vi "Goal_Clamp_on_Move.vi"(10 "Numeric":i32, 11 "60 Goal?":bool) -> ()   [LabVIEW 2012, in "Serenity_mk2.lvrbt"]
uses:
  Serenity_mk2.lvrbt
  <vilib>/NXT/Hardware/Plugins/Tetrix 180 deg Servo/Tetrix180ServoAddress.ctl
  <vilib>/NXT/NXTIO Xnodes/NXTIONodeSubVIs/TETRIX IO Move Servos.vi
  <vilib>/NXT/Subs/LVHSConnector.ctl
  <vilib>/NXT/NXTIO Xnodes/AddressXNode/NXTIOAddress.xnode
  <vilib>/NXT/NXTIO Xnodes/NXTIOXNode/NXTIO.xnode
  <vilib>/NXT/LegoClasses/BrickReference/BrickReference.lvclass
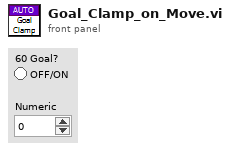
[diagram p1: front panel]
types:
  T1 = typedef "Tetrix180ServoAddress.ctl" = i32
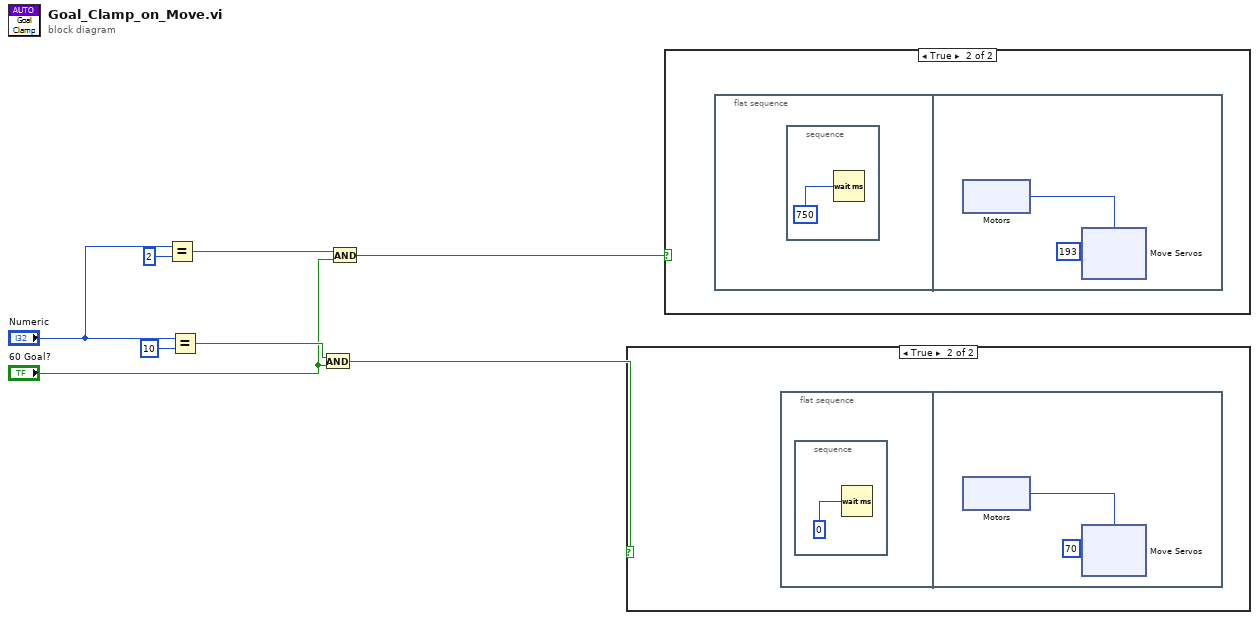
[diagram p0: block diagram]
diagram:
  n1 = Equal?(x="Numeric", y=2) -> (x = y?=w3:bool)
  n2 = Equal?(x="Numeric", y=10) -> (x = y?=w7:bool)
  n3 = And(x=w7, y="60 Goal?") -> (x .and. y?=w8:bool)
  n4 = And(x=w3, y="60 Goal?") -> (x .and. y?=w4:bool)
  n5 = case shown="True" w8 {
    frame False {
    }
    frame True {
      n6 = flat-sequence {
        frame #0 {
          n7 = stacked-sequence {
            frame #0 {
              n8 = Wait (ms)(milliseconds to wait=u32 0 ("Time (1 sec)")) -> ()  [unwired: 1 out]
            }
          }
        }
        frame #1 {
          n9 = xnode "Motors"() -> ("Motor"=w10:T1)
          n10 = xnode "Move Servos"("Position 1"=u8 70, "Motors"=w10) -> ()  [unwired: 1 in, 1 out]
        }
      }
    }
  }
  n11 = case shown="True" w4 {
    frame False {
    }
    frame True {
      n12 = flat-sequence {
        frame #0 {
          n13 = stacked-sequence {
            frame #0 {
              n14 = Wait (ms)(milliseconds to wait=u32 750 ("Time (1 sec)")) -> ()  [unwired: 1 out]
            }
          }
        }
        frame #1 {
          n15 = xnode "Motors"() -> ("Motor"=w21:T1)
          n16 = xnode "Move Servos"("Position 1"=u8 193, "Motors"=w21) -> ()  [unwired: 1 in, 1 out]
        }
      }
    }
  }
